vi "disconnect from library.vi"() -> ()   [LabVIEW 2025]
doc: "This module set some VIs Properties programaticaly.\n\nVI Properties:\nGeneral\n Separate compiled code from source = TRUE\nExecution\n Allow debugging = FALSE\n Reentrancy = Non-reentrant execution\n Prefered Execution System = instrument I/O\n Enable automatic error handling = FALSE"
panel:
  in  "Folder VIs Path":path
  # "This module set some VIs Properties programmaticaly.\n\nVI Methods:\nDisconnectFromLibrary\n\nVI Properties:\nGeneral\n\t            Separate compiled code from source = TRUE\nExecution\n\t             Allow debugging = FALSE\n\t             Reentrancy = Non-reentrant execution\n\t             Prefered Execution System = instrument I/O\n\t             Enable automatic error handling = FALSE"
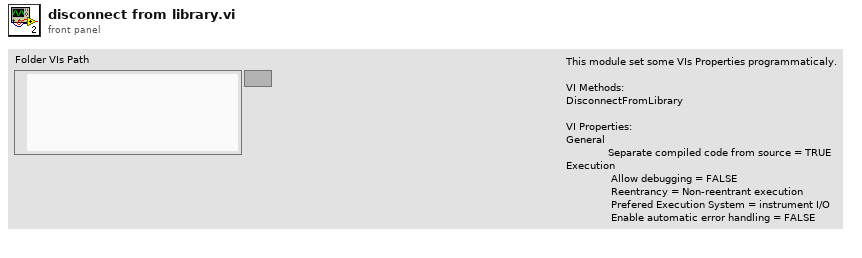
[diagram p1: front panel]
types:
  T1 = enum32{"invalid execution system", "user interface", "standard", "instrument i/o", "data acquisition", "other 1", "other 2", "same as caller"}
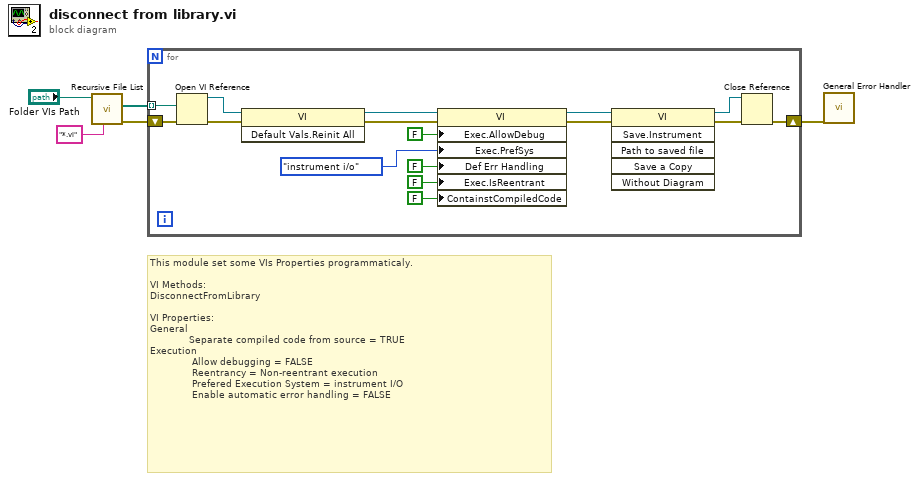
[diagram p0: block diagram]
diagram:
  # "This module set some VIs Properties programmaticaly.\n\nVI Methods:\nDisconnectFromLibrary\n\nVI Properties:\nGeneral\n\t            Separate compiled code from source = TRUE\nExecution\n\t             Allow debugging = FALSE\n\t             Reentrancy = Non-reentrant execution\n\t             Prefered Execution System = instrument I/O\n\t             Enable automatic error handling = FALSE"
  n1 = call <vilib>:"Recursive File List.vi"("pattern"="*.vi", "Folder Path"="Folder VIs Path") -> ("error out"=w3:errorcluster, "All Files in Dir"=w4:path[])  [unwired: 5 in, 3 out]
  n2 = for {
    tunnel: w4 -> [w21] mode=indexing
    shift-right: [w19] -> w2
    shift-left: w3 -> [w20]
    n3 = Open VI Reference(vi path=w21, error in (no error)=w20) -> (vi reference=w13:refnum<vi>, error out=w12:errorcluster)  [unwired: 4 in]
    n4 = invoke class="VI" method="Default Vals.Reinit All"(reference=w13, error in=w12) -> (reference out=w10:refnum<vi>, error out=w11:errorcluster)  [unwired: 1 in, 1 out]
    n5 = property class="VI"(reference=w10, error in=w11, "Exec.AllowDebug"=FALSE ("Execution:Allow Debugging"), "Exec.PrefSys"=T1."instrument i/o" ("Execution:Preferred Exec System"), "Def Err Handling"=FALSE ("Automatic Error Handling"), "Exec.IsReentrant"=FALSE ("Execution:Is Reentrant"), "ContainstCompiledCode"=FALSE ("Contains Compiled Code")) -> (reference out=w14:refnum<vi>, error out=w15:errorcluster)
    n6 = invoke class="VI" method="Save.Instrument"(reference=w14, error in=w15) -> (reference out=w17:refnum<vi>, error out=w18:errorcluster)  [unwired: 4 in, 4 out]
    n7 = Close Reference(reference=w17, error in (no error)=w18) -> (error out=w19:errorcluster)
  }
  n8 = call <vilib>:"General Error Handler.vi"("error in (no error)"=w2) -> ()  [unwired: 10 in, 5 out]
